vi "test_Split DMA by Direction.vi"(8 "error in (no error)":errorcluster) -> (0 "error out":errorcluster)   [LabVIEW 2019, in "Load And Parse Bitfile Testing.lvclass"]
uses:
  Load And Parse Bitfile Testing.lvclass
  Addon/Addon Shared/Types/DMA Information.ctl
  Addon/Addon Shared/Types/Data Type.ctl
  <vilib>/addons/_JKI Toolkits/VI Tester/TestCase.llb/TestCase.lvclass
  Addon/Addon System Explorer/FPGA Addon System Explorer.lvlib
  Addon/Addon Shared/FPGA Addon Shared.lvlib
  C:/Program Files (x86)/National Instruments/LabVIEW 2019/vi.lib/addons/_JKI Toolkits/VI Tester/TestCase.llb/TestCase.lvclass
panel:
  out "TestCase out":refnum<class "Load And Parse Bitfile Testing.lvclass">
  in  "TestCase in":refnum<class "Load And Parse Bitfile Testing.lvclass">
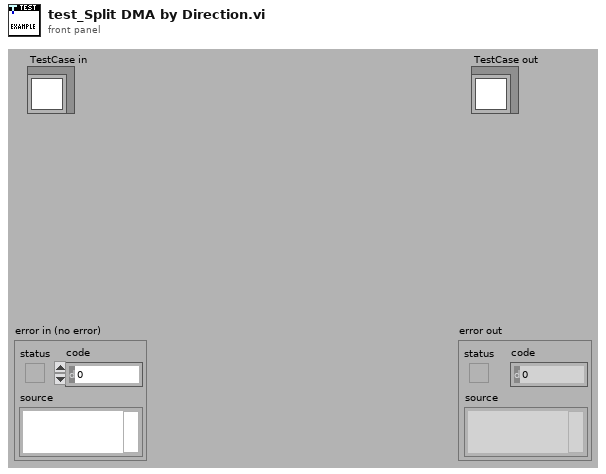
[diagram p1: front panel]
types:
  T1 = typedef "FPGA Addon Shared.lvlib/DMA Information.ctl" = cluster{"Name":string, "Data Type":T2}
  T2 = typedef "FPGA Addon Shared.lvlib/Data Type.ctl" = enum8{"<Null>", "I8", "I16", "I32", "I64", "U8", "U16", "U32", "U64", "SGL", "Boolean", "Analog PWM In Settings", "Analog PWM In", "Digital PWM In Settings", "Digital PWM In", "Digital PWM Out", "Sine Out", "FXP+/-24.5", "FXP+/-16.5", "FXP+/-32.8", "FXP+/-64.32", "FXP+/-16.7", "FXP+/-20.5", "FXP+/-27.5", "FXP+/-32.16", "FXP+16.3", "FXP+18.3", "Digital Static In", "Digital Static Out", "Digital Static In Settings", "Digital WSS Out", "Quad Encoder Settings", "Quad Encoder In", "Group"}
  T3 = typedef "Fifo_DMA_Config.ctl" = cluster{"Name":string, "Depth":u32, "Write? (Deprecated:Use Implementation)":bool, "Physical Channel":u32, "Base Address":u32, "Data Width":u32, "Data Type":T4, "FXP Properties":variant, "Write Window Address":u32, "Implementation":T5, "Control Set":u32}
  T4 = typedef "niFpgaDataTypeControl.ctl" = enum32{"Boolean", "I8", "I16", "I32", "I64", "U8", "U16", "U32", "U64", "FXP", "CustomControl", "SGL"}
  T5 = typedef "niFpgaDmaChannelImplementation.ctl" = enum16{"niFpgaTargetToHost", "niFpgaHostToTarget", "niFpgaPeerToPeerWriter", "niFpgaPeerToPeerReader", "niCoreTargetToHost", "niCoreHostToTarget"}
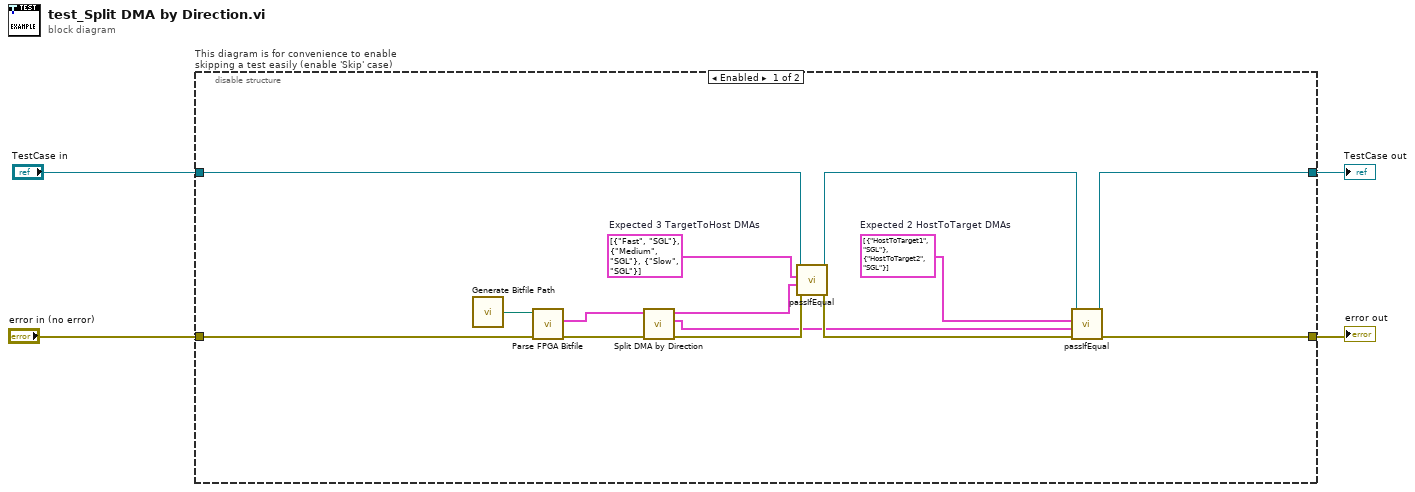
[diagram p0: block diagram]
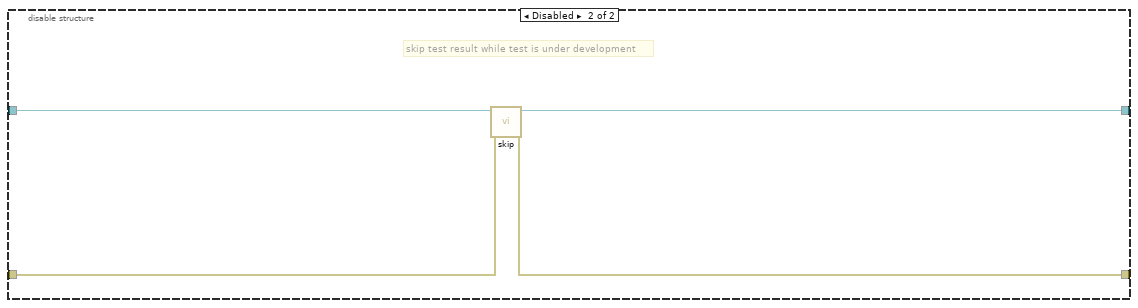
[diagram p2: hidden frame]
diagram:
  n1 = disable-structure "This diagram is for convenience to enable skipping a test easily (enable 'Skip' case)" shown="Enabled" {
    disable-tunnel: "TestCase in" -> [w18 w22]
    disable-tunnel: [w8 w20] -> w1
    disable-tunnel: [w9 w21] -> w3
    disable-tunnel: "error in (no error)" -> [w17 w19]
    frame Enabled {
      w7 = T1[] [{"Name"="HostToTarget1", "Data Type"=enum."SGL"}, {"Name"="HostToTarget2", "Data Type"=enum."SGL"}]  # Expected 2 HostToTarget DMAs
      w12 = T1[] [{"Name"="Fast", "Data Type"=enum."SGL"}, {"Name"="Medium", "Data Type"=enum."SGL"}, {"Name"="Slow", "Data Type"=enum."SGL"}]  # Expected 3 TargetToHost DMAs
      n2 = call "Generate Bitfile Path.vi"() -> ("Bitfile Path"=w5:path)
      n3 = call "Parse FPGA Bitfile.vi"("error in (no error)"=w17, "Path"=w5) -> ("error out"=w15:errorcluster, "DMA configuration array"=w16:T3[])  [unwired: 7 in, 1 out]
      n4 = call "Split DMA by Direction.vi"("error in"=w15, "DMA configuration array"=w16) -> ("error out"=w14:errorcluster, "HostToTarget"=w6:T1[], "TargetToHost"=w13:T1[])  [unwired: 7 in]
      n5 = call-dynamic "passIfEqual.vi"("error in (no error)"=w14, "y"=w13, "x"=w12, "TestCase in"=w18) -> ("error out"=w10:errorcluster, "TestCase out"=w11:refnum<class "Load And Parse Bitfile Testing.lvclass">)  [unwired: 6 in]
      n6 = call-dynamic "passIfEqual.vi"("error in (no error)"=w10, "y"=w6, "x"=w7, "TestCase in"=w11) -> ("error out"=w9:errorcluster, "TestCase out"=w8:refnum<class "Load And Parse Bitfile Testing.lvclass">)  [unwired: 6 in]
    }
    frame Disabled {
      # "skip test result while test is under development"
      n7 = call <vilib>:"skip.vi"("error in (no error)"=w19, "TestCase in"=w22) -> ("error out"=w21:errorcluster, "TestCase out"=w20:refnum<class "Load And Parse Bitfile Testing.lvclass">)  [unwired: 8 in]
    }
  }
  "error out" <- w3
  "TestCase out" <- w1
